vi "CONFIG FALCON Climber.vi"(8 "error in (no error)":errorcluster, 10 "PhoenixMotorControlDevRef in":T3, 11 "ARM Climber range":T8) -> (0 "error out":errorcluster, 3 "PhoenixMotorControlDevRef out":T3)   [LabVIEW 2020]
uses:
  <vilib>/Rock Robotics/WPI/MotorControl/WPI_MotorControlDeviceRef.ctl
  <vilib>/Rock Robotics/WPI/MotorControl/WPI_MotorControlType.ctl
  <vilib>/Rock Robotics/SystemInterfaces/DIO/FPGA_DIOPWMChannel.ctl
  <vilib>/Rock Robotics/WPI/PWM/WPI_PWMDeadband.ctl
  <vilib>/Rock Robotics/SystemInterfaces/DIO/FPGA_DIOChannel.ctl
  <vilib>/Rock Robotics/WPI/ThirdParty/Phoenix-LabVIEW/Motor Controller/Controls/CTRE_Phoenix_MotorControl_LimitSwitchSource_Local.ctl
  <vilib>/Rock Robotics/WPI/ThirdParty/Phoenix-LabVIEW/Motor Controller/Controls/CTRE_Phoenix_MotorControl_LimitSwitchNormal.ctl
panel:
  in  "REV Limit Switch Source":T1
  in  "REV NormallyOpenOrClosed":T2
  in  "FWD NormallyOpenOrClosed":T2
  in  "FWD Limit Switch Source":T1
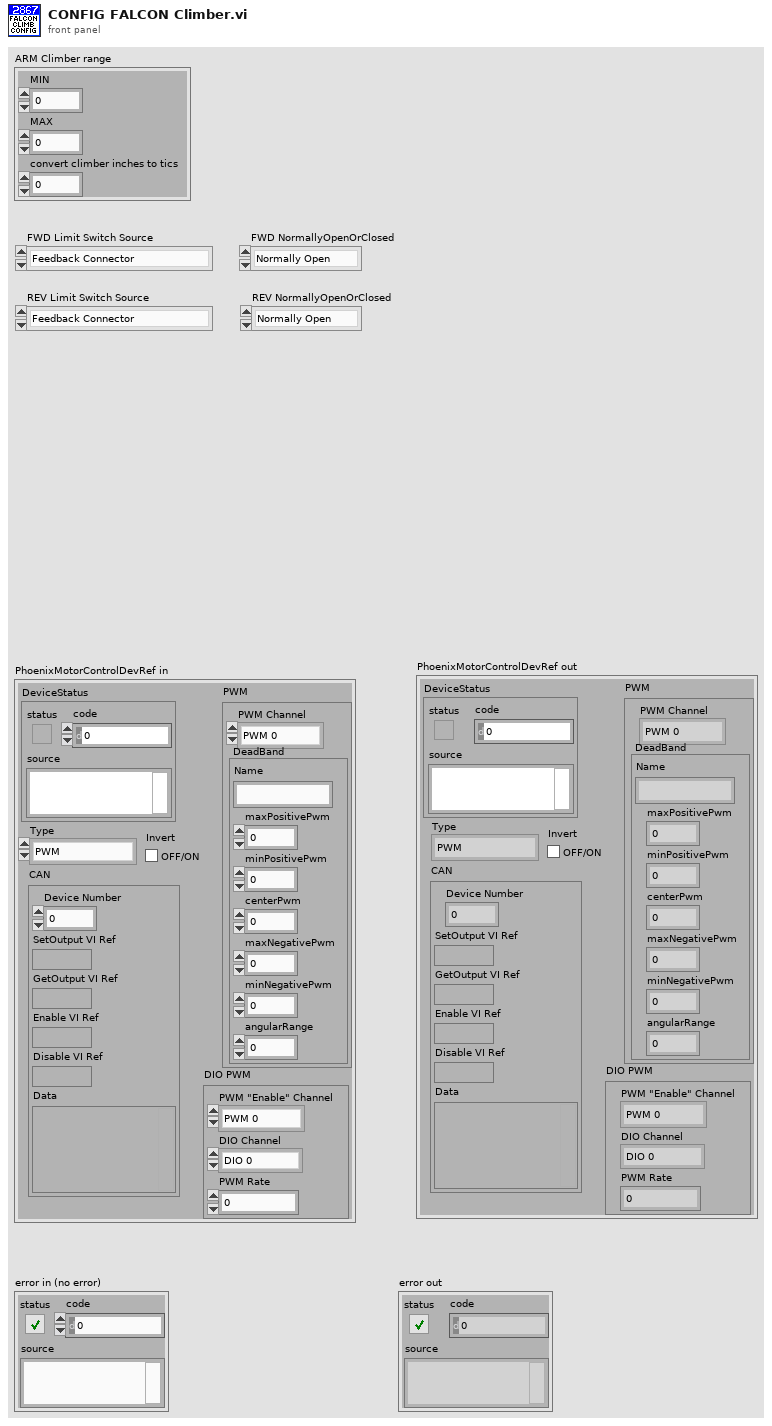
[diagram p1: front panel]
types:
  T1 = typedef "CTRE_Phoenix_MotorControl_LimitSwitchSource_Local.ctl" = enum16{"Feedback Connector", "Remote Talon SRX", "Remote CANifier", "Deactivated"}
  T2 = typedef "CTRE_Phoenix_MotorControl_LimitSwitchNormal.ctl" = enum16{"Normally Open", "Normally Closed", "Disabled"}
  T3 = typedef "WPI_MotorControlDeviceRef.ctl" = cluster{"DeviceStatus":errorcluster, "Type":T4, "PWM":cluster{"PWM Channel":T5, "DeadBand":T6}, "CAN":cluster{"Device Number":u8, "SetOutput VI Ref":variant, "GetOutput VI Ref":variant, "Enable VI Ref":variant, "Disable VI Ref":variant, "Data":variant}, "Invert":bool, "DIO PWM":cluster{"PWM \"Enable\" Channel":T5, "DIOChannel":T7, "PWM Rate":dbl}}
  T4 = typedef "WPI_MotorControlType.ctl" = enum16{"PWM", "CAN", "DIO PWM"}
  T5 = typedef "FPGA_DIOPWMChannel.ctl" = enum8{"PWM 0", "PWM 1", "PWM 2", "PWM 3", "PWM 4", "PWM 5", "PWM 6", "PWM 7", "PWM 8", "PWM 9", "PWM MXP 0", "PWM MXP 1", "PWM MXP 2", "PWM MXP 3", "PWM MXP 4", "PWM MXP 5", "PWM MXP 6", "PWM MXP 7", "PWM MXP 8", "PWM MXP 9", "Invalid"}
  T6 = typedef "WPI_PWMDeadband.ctl" = cluster{"Name":string, "maxPositivePwm":i32, "minPositivePwm":i32, "centerPwm":i32, "maxNegativePwm":i32, "minNegativePwm":i32, "angularRange":u16}
  T7 = typedef "FPGA_DIOChannel.ctl" = enum8{"DIO 0", "DIO 1", "DIO 2", "DIO 3", "DIO 4", "DIO 5", "DIO 6", "DIO 7", "DIO 8", "DIO 9", "DIO MXP 0", "DIO MXP 1", "DIO MXP 2", "DIO MXP 3", "DIO MXP 4", "DIO MXP 5", "DIO MXP 6", "DIO MXP 7", "DIO MXP 8", "DIO MXP 9", "DIO MXP 10", "DIO MXP 11", "DIO MXP 12", "DIO MXP 13", "DIO MXP 14", "DIO MXP 15", "SPI Port CS1", "SPI Port CS2", "SPI Port CS3", "SPI Port MISO", "SPI Port MOSI", "Invalid"}
  T8 = cluster{"MIN":dbl, "MAX":dbl, "convert climber inches to tics":dbl}
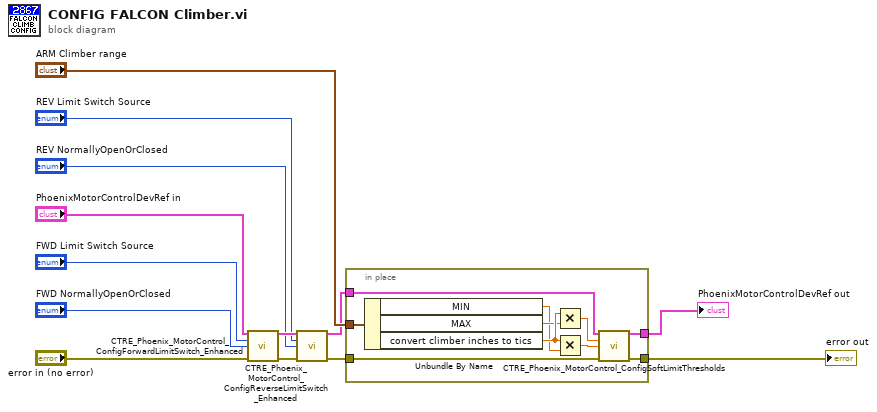
[diagram p0: block diagram]
diagram:
  n1 = call <vilib>:"CTRE_Phoenix_MotorControl_ConfigForwardLimitSwitch_Enhanced.vi"("PhoenixMotorControlDevRef"="PhoenixMotorControlDevRef in", "Limit Switch Source"="FWD Limit Switch Source", "NormallyOpenOrClosed"="FWD NormallyOpenOrClosed", "error in (no error)"="error in (no error)") -> ("PhoenixMotorControlDevRef"=w7:T3, "error out"=w5:errorcluster)  [unwired: 10 in]
  n2 = call <vilib>:"CTRE_Phoenix_MotorControl_ConfigReverseLimitSwitch_Enhanced.vi"("PhoenixMotorControlDevRef"=w7, "Limit Switch Source"="REV Limit Switch Source", "NormallyOpenOrClosed"="REV NormallyOpenOrClosed", "error in (no error)"=w5) -> ("PhoenixMotorControlDevRef"=w8:T3, "error out"=w4:errorcluster)  [unwired: 10 in]
  n3 = in-place {
    in-place-border: "ARM Climber range" -> [w23]
    in-place-border: w8 -> [w22]
    in-place-border: [w21] -> w6
    in-place-border: w4 -> [w20]
    in-place-border: [w19] -> w3
    n4 = Unbundle By Name(w23) -> ("MIN"=w14:dbl, "MAX"=w15:dbl, "convert climber inches to tics"=w16:dbl)
    n5 = Multiply(x=w16, y=w15) -> (x*y=w17:dbl)
    n6 = Multiply(x=w16, y=w14) -> (x*y=w18:dbl)
    n7 = call <vilib>:"CTRE_Phoenix_MotorControl_ConfigSoftLimitThresholds.vi"("PhoenixMotorControlDevRef"=w22, "Forward Soft Limit"=w17, "Reverse Soft Limit"=w18, "error in (no error)"=w20) -> ("PhoenixMotorControlDevRef"=w21:T3, "error out"=w19:errorcluster)  [unwired: 10 in]
  }
  "error out" <- w3
  "PhoenixMotorControlDevRef out" <- w6
